vi "Pod Code.vi"() -> ()   [LabVIEW 2017]
uses:
  Type Defs/Relays.ctl
  Type Defs/tempReadings.ctl
  Sensors/Power Sensor - Adafruit INA219/INA219 Measurements.ctl
  Type Defs/telemetryReading.ctl
  <vilib>/Utility/RT CPU Load.ctl
  Type Defs/PodState.ctl
  Type Defs/tofReading.ctl
  Type Defs/pressureReading.ctl
  Type Defs/allLaserReadings.ctl
  Type Defs/laserReading.ctl
  Type Defs/AnalogPressureReading.ctl
  Type Defs/criticalTelemetry.ctl
  Sensors/Time of Flight - VL6180/VL6180 Resource.ctl
  Sensors/Power Sensor - Adafruit INA219/INA219 Config Options.ctl
  Type Defs/thermopileSettings.ctl
  Sensors/Pressure Sensor - BMP180/BMP180 Config Options.ctl
  Type Defs/SensorStates.ctl
  Type Defs/allData.ctl
  <vilib>/Platform/TimedLoop/XDataNode/timing_clust.ctl
  <vilib>/Platform/TimedLoop/XDataNode/nitl_modes.ctl
  <vilib>/Platform/TimedLoop/XDataNode/wakeup.ctl
  <vilib>/myRIO/Instrument Drivers/Onboard IO/DIO/typedefs/DIO Reference.ctl
  <vilib>/myRIO/Common/Instrument Driver Framework/Utilities/typedefs/myRIO Generic Hardware Reference.ctl
  <vilib>/myRIO/Common/Instrument Driver Framework/Utilities/typedefs/Hardware Version Enum.ctl
  <vilib>/myRIO/Common/Instrument Driver Framework/Utilities/typedefs/myRIO v1.0 Reference.ctl
  <vilib>/myRIO/Common/Instrument Driver Framework/Utilities/typedefs/Generic FPGA Reference.ctl
  <vilib>/myRIO/Common/Instrument Driver Framework/myRIO v1.0/DIO/typedefs/DIO Channels List.ctl
  <vilib>/myRIO/Common/Instrument Driver Framework/myRIO v1.0/DIO/typedefs/DIO Channels Enum.ctl
  <vilib>/userdefined/High Color/nirio_resource_hc.ctl
  <vilib>/myRIO/Common/Instrument Driver Framework/Utilities/vis/Is FPGA Ref Available.vi
  <vilib>/myRIO/Common/Instrument Driver Framework/myRIO v1.0/DIO/vis/myRIO v1.1 Open DIO.vi
  <vilib>/myRIO/Instrument Drivers/Onboard IO/DIO/vis/Read.vi
  <vilib>/myRIO/Instrument Drivers/Onboard IO/DIO/vis/Write.vi
  <vilib>/myRIO/Common/Instrument Driver Framework/Utilities/vis/Validate Channels.vi
  <vilib>/myRIO/Common/Instrument Driver Framework/myRIO v1.0/DIO/vis/myRIO v1.0 Reserve DIO.vi
  <vilib>/myRIO/Common/Instrument Driver Framework/myRIO v1.0/Resource Manager/vis/myRIO v1.0 Reserve Channel List.vi
  <vilib>/myRIO/Common/Instrument Driver Framework/myRIO v1.0/DIO/vis/myRIO v1.0 Build MUX Configuration DIO.vi
  <vilib>/myRIO/Common/Instrument Driver Framework/myRIO v1.0/Resource Manager/vis/myRIO v1.0 Reserve Channel.vi
  <vilib>/myRIO/Common/Instrument Driver Framework/myRIO v1.0/Resource Manager/vis/myRIO v1.0 Unreserve Channel.vi
  <vilib>/myRIO/Common/Instrument Driver Framework/myRIO v1.0/Resource Manager/vis/myRIO v1.0 Create Configuration List.vi
  <vilib>/myRIO/Common/Instrument Driver Framework/myRIO v1.0/Resource Manager/vis/myRIO v1.0 Build Mutex Name.vi
  <vilib>/Utility/VariantDataType/GetNumericInfo.vi
  <vilib>/Utility/error.llb/Error Cluster From Error Code.vi
  <vilib>/myRIO/Common/Instrument Driver Framework/myRIO v1.0/myRIO v1.1 Open.vi
  <vilib>/myRIO/Common/Instrument Driver Framework/Utilities/vis/IO Manager.vi
  <vilib>/myRIO/Common/Instrument Driver Framework/Utilities/vis/Configuration Manager.vi
  <vilib>/myRIO/Common/Instrument Driver Framework/myRIO v1.0/Resource Manager/vis/myRIO v1.0 Configure IO.vi
  <vilib>/myRIO/Common/Instrument Driver Framework/myRIO v1.0/myRIO v1.0 Close.vi
  <vilib>/myRIO/Common/Instrument Driver Framework/myRIO v1.0/DIO/vis/myRIO v1.0 Write DIO.vi
  <vilib>/myRIO/Common/Instrument Driver Framework/myRIO v1.0/DIO/vis/myRIO v1.0 Read DIO.vi
  <vilib>/myRIO/Express VI/Onboard IO/DO/DO Express VI.xnode
  <vilib>/myRIO/Instrument Drivers/Onboard IO/DIO/vis/myRIO DIO Open.xnode
  <vilib>/platform/TimedLoop/XDataNode/XDataNode.xnode
  <vilib>/myRIO/Express VI/Onboard IO/DI/DI Express VI.xnode
  <vilib>/myRIO/Instrument Drivers/Onboard IO/DIO/DIO.lvlib
  <vilib>/Platform/TimedLoop/XDataNode/XDNodeRunTimeDep.lvlib
  <vilib>/NI_Real-Time Target Support.lvlib
panel:
  out "Data Snap Period":u32
  out "Slow Sensor Period":u32
  out "State Machine Period":u32
  out "Fast Sensor Period":u32
  out "Actuators":u32
  out "Latest Critical Telemetry":T1
  out "Analog Pressure Reading":T3
  out "Laser Error":errorcluster
  out "Laser Readings":T4
  out "Pressure Reading":T6
  out "ToF Readings":T7[](array[typedef])
  out "Pod State":T2
  in  "Logging":bool
  out "Sensor Error 2":errorcluster
  out "# elements in queue":i32
  out "CPU loads":T8[](array[typedef]) {"ISR (%)" format="%#.2f"; "Idle (%)" format="%#.2f"; "Background (%)" format="%#.2f"; "Normal (%)" format="%#.2f"; "Above Normal (%)" format="%#.2f"; "High (%)" format="%#.2g"; "Timed Structures (%)" format="%#.2g"; "Time Critical (%)" format="%#.2g"; "Total (%)" format="%#.2g"}
  out "Log":T9[][](array[typedef])
  in  "Power I2C Addrs":u8[](array[numeric])=[68, 65, 69] format="%.0x"
  out "Power Readings":T10[](array[typedef]) {"Current" format="%#.3g A"; "Power" format="%#.3g W"; "Shunt Voltage" format=" %#.3g V"; "Bus Voltage" format="%#.3g V"; "Voltage (Total)" format="%#.3g V"}
  out "ThermalReadings":T11[](array[typedef]) {"Ambient Temp (°F)" format="%.2f °F"; "Ambient Temp (°C)" format="%.2f °C"; "Object Temp (°F)" format="%.2f °F"; "Object Temp (°C)" format="%.2f °C"}
  in  "Thermal I2C Addrs":u8[](array[numeric])=[64, 67] format="%.0x"
  in  "Reset Count":bool
  in  "ToFs in use":T12[](array[typedef])=[enum."ToF1", enum."ToF2", enum."ToF3", enum."ToF4"]
  out "Sensor Error":errorcluster
  in  "Reset Sensors":bool
  out "State Error":errorcluster
  in  "Stop Button":bool
  # "Config"
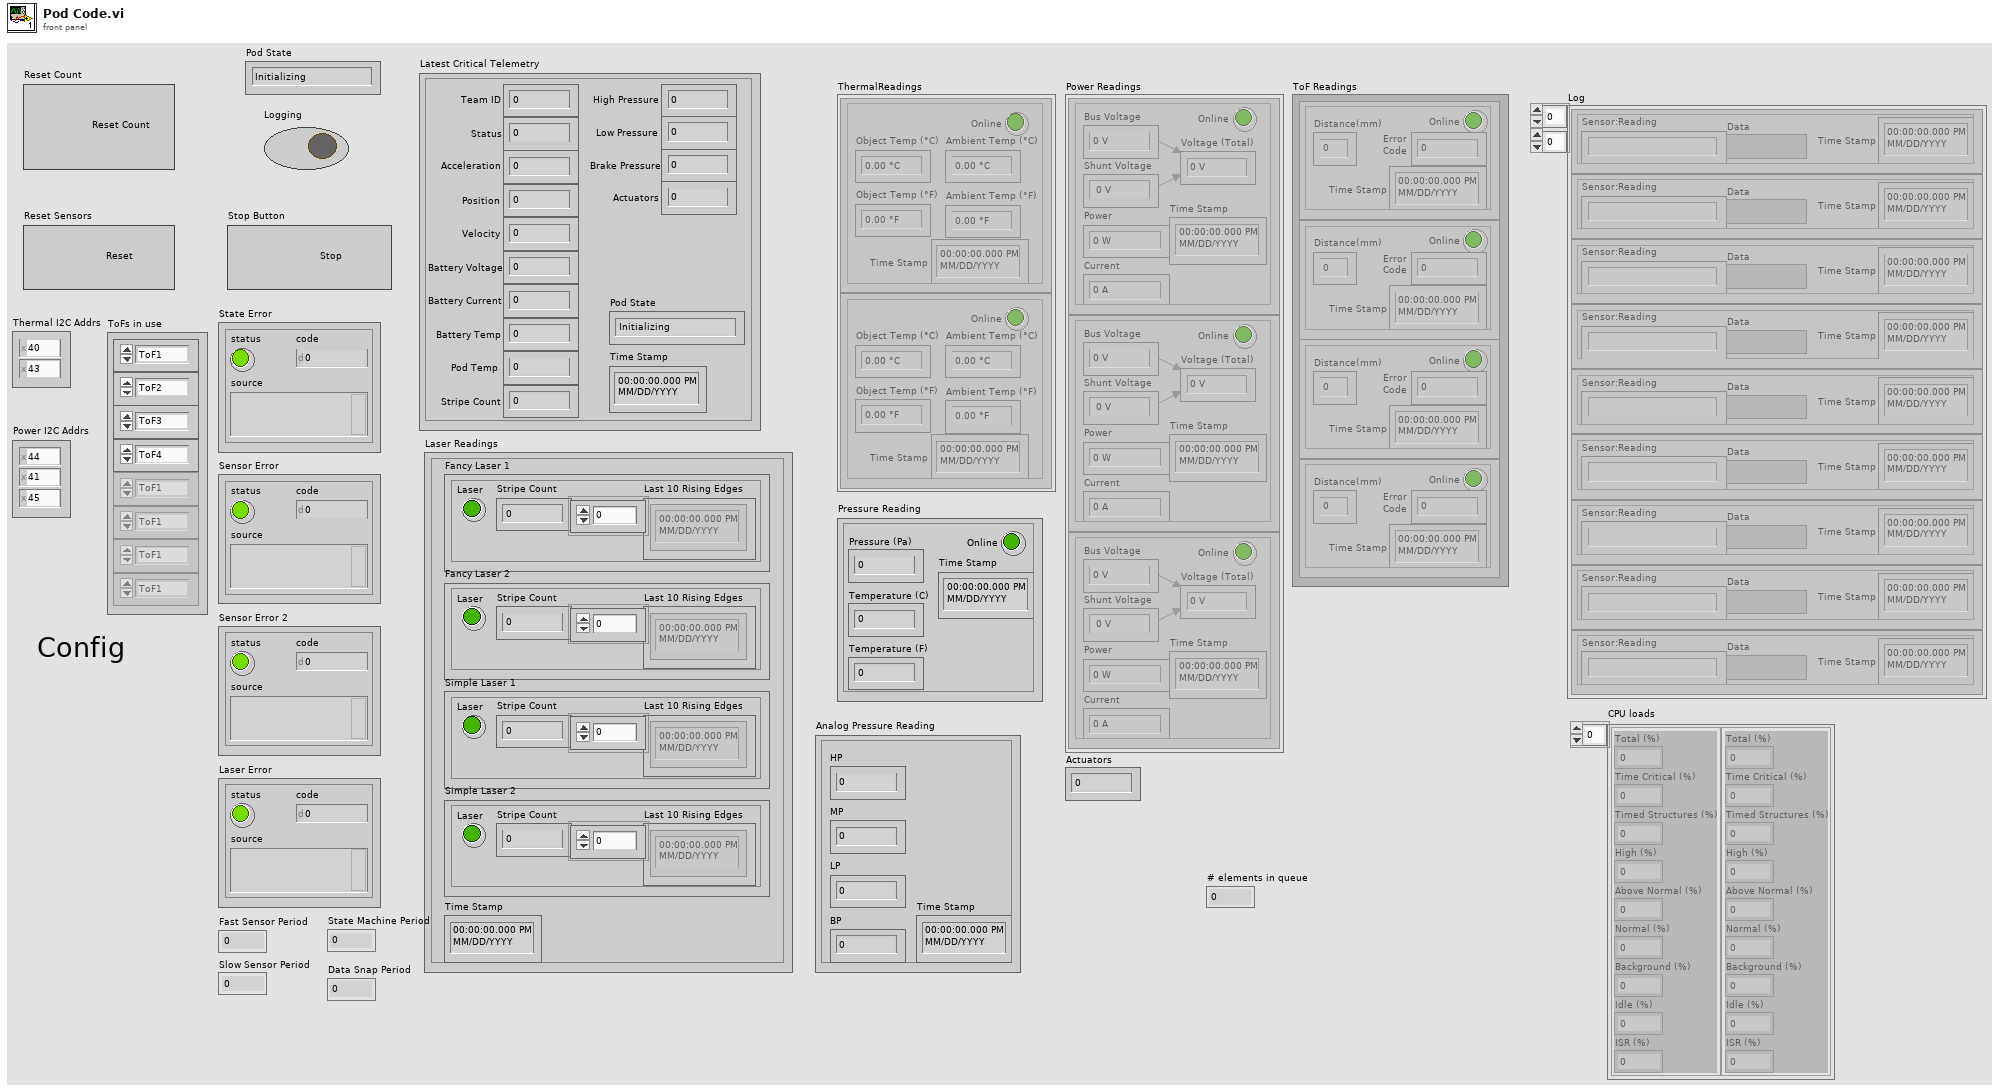
[diagram p1: front panel]
types:
  T1 = typedef "criticalTelemetry.ctl" = cluster{"Team ID":u8, "Status":u8, "Acceleration":i32, "Position":i32, "Velocity":i32, "Battery Voltage":i32, "Battery Current":i32, "Battery Temp":i32, "Pod Temp":i32, "Stripe Count":u32, "High Pressure":dbl, "Low Pressure":dbl, "Brake Pressure":dbl, "Actuators":u32, "Pod State":T2, "Time Stamp":timestamp}
  T2 = typedef "PodState.ctl" = enum16{"Initializing", "Pre-flight Testing", "Ready", "Pushing", "Coast", "Braking", "Post-flight", "Fault"}
  T3 = typedef "AnalogPressureReading.ctl" = cluster{"HP":dbl, "MP":dbl, "LP":dbl, "BP":dbl, "Time Stamp":timestamp}
  T4 = typedef "allLaserReadings.ctl" = cluster{"Fancy Laser 1":T5, "Fancy Laser 2":T5, "Simple Laser 1":T5, "Simple Laser 2":T5, "Time Stamp":timestamp}
  T5 = typedef "laserReading.ctl" = cluster{"Laser":bool, "Stripe Count":u32, "Last 10 Rising Edges":timestamp[]}
  T6 = typedef "pressureReading.ctl" = cluster{"Time Stamp":timestamp, "Online":bool, "Temperature (C)":dbl, "Pressure (Pa)":dbl, "Temperature (F)":dbl}
  T7 = typedef "tofReading.ctl" = cluster{"Distance(mm)":u8, "Online":bool, "Error\nCode":u8, "Time Stamp":timestamp}
  T8 = typedef "NI_Real-Time Target Support.lvlib/RT CPU Load.ctl" = cluster{"Total (%)":dbl, "Time Critical (%)":dbl, "Timed Structures (%)":dbl, "High (%)":dbl, "Above Normal (%)":dbl, "Normal (%)":dbl, "Background (%)":dbl, "Idle (%)":dbl, "ISR (%)":dbl}
  T9 = typedef "telemetryReading.ctl" = cluster{"Sensor:Reading":string, "Data":variant, "Time Stamp":timestamp}
  T10 = typedef "INA219 Measurements.ctl" = cluster{"Voltage (Total)":dbl, "Bus Voltage":dbl, "Shunt Voltage":dbl, "Power":dbl, "Current":dbl, "Online":bool, "Time Stamp":timestamp}
  T11 = typedef "tempReadings.ctl" = cluster{"Object Temp (°C)":dbl, "Object Temp (°F)":dbl, "Ambient Temp (°C)":dbl, "Ambient Temp (°F)":dbl, "Online":bool, "Time Stamp":timestamp}
  T12 = typedef "Relays.ctl" = enum16{"ToF1", "ToF2", "ToF3", "ToF4", "ToF5", "ToF6", "ToF7", "ToF8", "SensePwr", "All"}
  T13 = typedef "SensorStates.ctl" = enum16{"Reset", "Read", "Close"}
  T14 = typedef "BMP180 Config Options.ctl" = cluster{"I2C":cluster{"Slave Address":u8, "Channel":u8}, "Mode":enum8{"Ultra Low Power", "Standard", "High Resolution", "Ultra High Resolution"}, "Cal Coefs":cluster{"AC1":cluster{"Addr:":u8, "Val:":u16}, "AC2":cluster{"Addr:":u8, "Val:":u16}, "AC3":cluster{"Addr:":u8, "Val:":u16}, "AC4":cluster{"Addr:":u8, "Val:":u16}, "AC5":cluster{"Addr:":u8, "Val:":u16}, "AC6":cluster{"Addr:":u8, "Val:":u16}, "B1":cluster{"Addr:":u8, "Val:":u16}, "B2":cluster{"Addr:":u8, "Val:":u16}, "MB":cluster{"Addr:":u8, "Val:":u16}, "MC":cluster{"Addr:":u8, "Val:":u16}, "MD":cluster{"Addr:":u8, "Val:":u16}}, "Online":bool}
  T15 = typedef "thermopileSettings.ctl" = cluster{"Online":bool, "I2C Channel":u8, "I2C Slave Address":u8, "Valid Sample":bool, "Samples to Average":u16, "Last Temp Readings":T11, "Last Reading Time":dbl, "Last Conv Time":dbl}
  T16 = typedef "INA219 Config Options.ctl" = cluster{"I2C":cluster{"Slave Address":u8, "Channel":u8}, "Reset bit":u8, "Bus Voltage Range":u8, "PGA/Shunt Voltage Gain":u8, "Bus Voltage ADC Settings":u8, "Shunt Voltage ADC Settings":u8, "Mode":u8, "Calibration Value":u16, "Online":bool, "Shunt Resistor":dbl}
  T17 = typedef "VL6180 Resource.ctl" = cluster{"I2C Channel":u8, "I2C Slave Address":u8, "Online":bool}
  T18 = typedef "XDNodeRunTimeDep.lvlib/timing_clust.ctl" = cluster{"Expected End [f-1]":u64, "Actual End [f-1]":u64, "Finished Late? [f-1]":bool, "Expected End [i-1]":u64, "Actual End [i-1]":u64, "Finished Late? [i-1]":bool, "Expected Start [i]":u64, "Actual Start [i]":u64, "Expected Start [f]":u64, "Actual Start [f]":u64, "Source Name":string, "Structure Name":string, "Period":i64, "Deadline":i64, "Offset":i64, "Start":i64, "Priority":i32, "Timeout":i32, "Mode":T19, "Wakeup Reason":T20, "Error":errorcluster, "Source Type":string, "Secondary Source Type":string, "Global End Time":u64, "Global Start Time":u64, "Frame Duration":u64, "Iteration Duration":u64, "Assigned CPU":i32, "I/O Scan Engine Mode":u32}
  T19 = typedef "XDNodeRunTimeDep.lvlib/nitl_modes.ctl" = enum32{"No Change", "Process missed periods, maintain original phase", "Discard missed periods, maintain original phase", "Process missed periods, ignore original phase", "Discard missed periods, ignore original phase"}
  T20 = typedef "XDNodeRunTimeDep.lvlib/wakeup.ctl" = enum32{"Normal", "Aborted", "Asynchronous wakeup", "Timing source error", "Timed loop error", "Timeout"}
  T21 = typedef "DIO.lvlib/DIO Reference.ctl" = cluster{"myRIO Reference":T22, "DIO Channels List":T26}
  T22 = typedef "myRIO Generic Hardware Reference.ctl" = cluster{"myRIO Model":T23, "myRIO Hardware Reference":T24}
  T23 = typedef "Hardware Version Enum.ctl" = enum16{"Unknown", "myRIO-1900", "myRIO-1950", "roboRIO", "NI ELVIS RIO CM"}
  T24 = typedef "myRIO v1.0 Reference.ctl" = cluster{"Generic FPGA Reference":T25, "Allow multiple opens":bool}
  T25 = typedef "Generic FPGA Reference.ctl" = refnum<k20>
  T26 = typedef "DIO Channels List.ctl" = T27[]
  T27 = typedef "DIO Channels Enum.ctl" = enum16{"Not Connected", "C/DIO0", "C/DIO1", "C/DIO2", "C/DIO3", "C/DIO4", "C/DIO5", "C/DIO6", "C/DIO7", "A/DIO0", "A/DIO1", "A/DIO2", "A/DIO3", "A/DIO4", "A/DIO5", "A/DIO6", "A/DIO7", "A/DIO8", "A/DIO9", "A/DIO10", "A/DIO11", "A/DIO12", "A/DIO13", "A/DIO14", "A/DIO15", "B/DIO0", "B/DIO1", "B/DIO2", "B/DIO3", "B/DIO4", "B/DIO5", "B/DIO6", "B/DIO7", "B/DIO8", "B/DIO9", "B/DIO10", "B/DIO11", "B/DIO12", "B/DIO13", "B/DIO14", "B/DIO15", "LED0", "LED1", "LED2", "LED3", "Button0", "DIO/DIO0", "DIO/DIO1", "DIO/DIO2", "DIO/DIO3", "DIO/DIO4", "DIO/DIO5", "DIO/DIO6", "DIO/DIO7", "DIO/DIO8", "DIO/DIO9", "SPI/CS0", "SPI/CS1", "SPI/CS2", "SPI/CS3", "LED RADIO (Green)", "LED RADIO (Red)", "LED COMM (Green)", "LED COMM (Red)", "LED MODE (Green)", "LED MODE (Red)"}
  T28 = typedef "nirio_resource_hc.ctl" = tag
  T29 = typedef "allData.ctl" = cluster{"Power Readings":T10[], "ThermalReadings":T11[], "Analog Pressure Reading":T3, "Laser Readings":T4, "Pod State":T2, "seconds since 1Jan1904":timestamp, "ToF Readings":T7[], "CPU loads":T8[], "Actuators":u32, "Pressure Reading":T6, "Laser Error":errorcluster, "Sensor Error":errorcluster, "Sensor Error 2":errorcluster, "State Error":errorcluster}
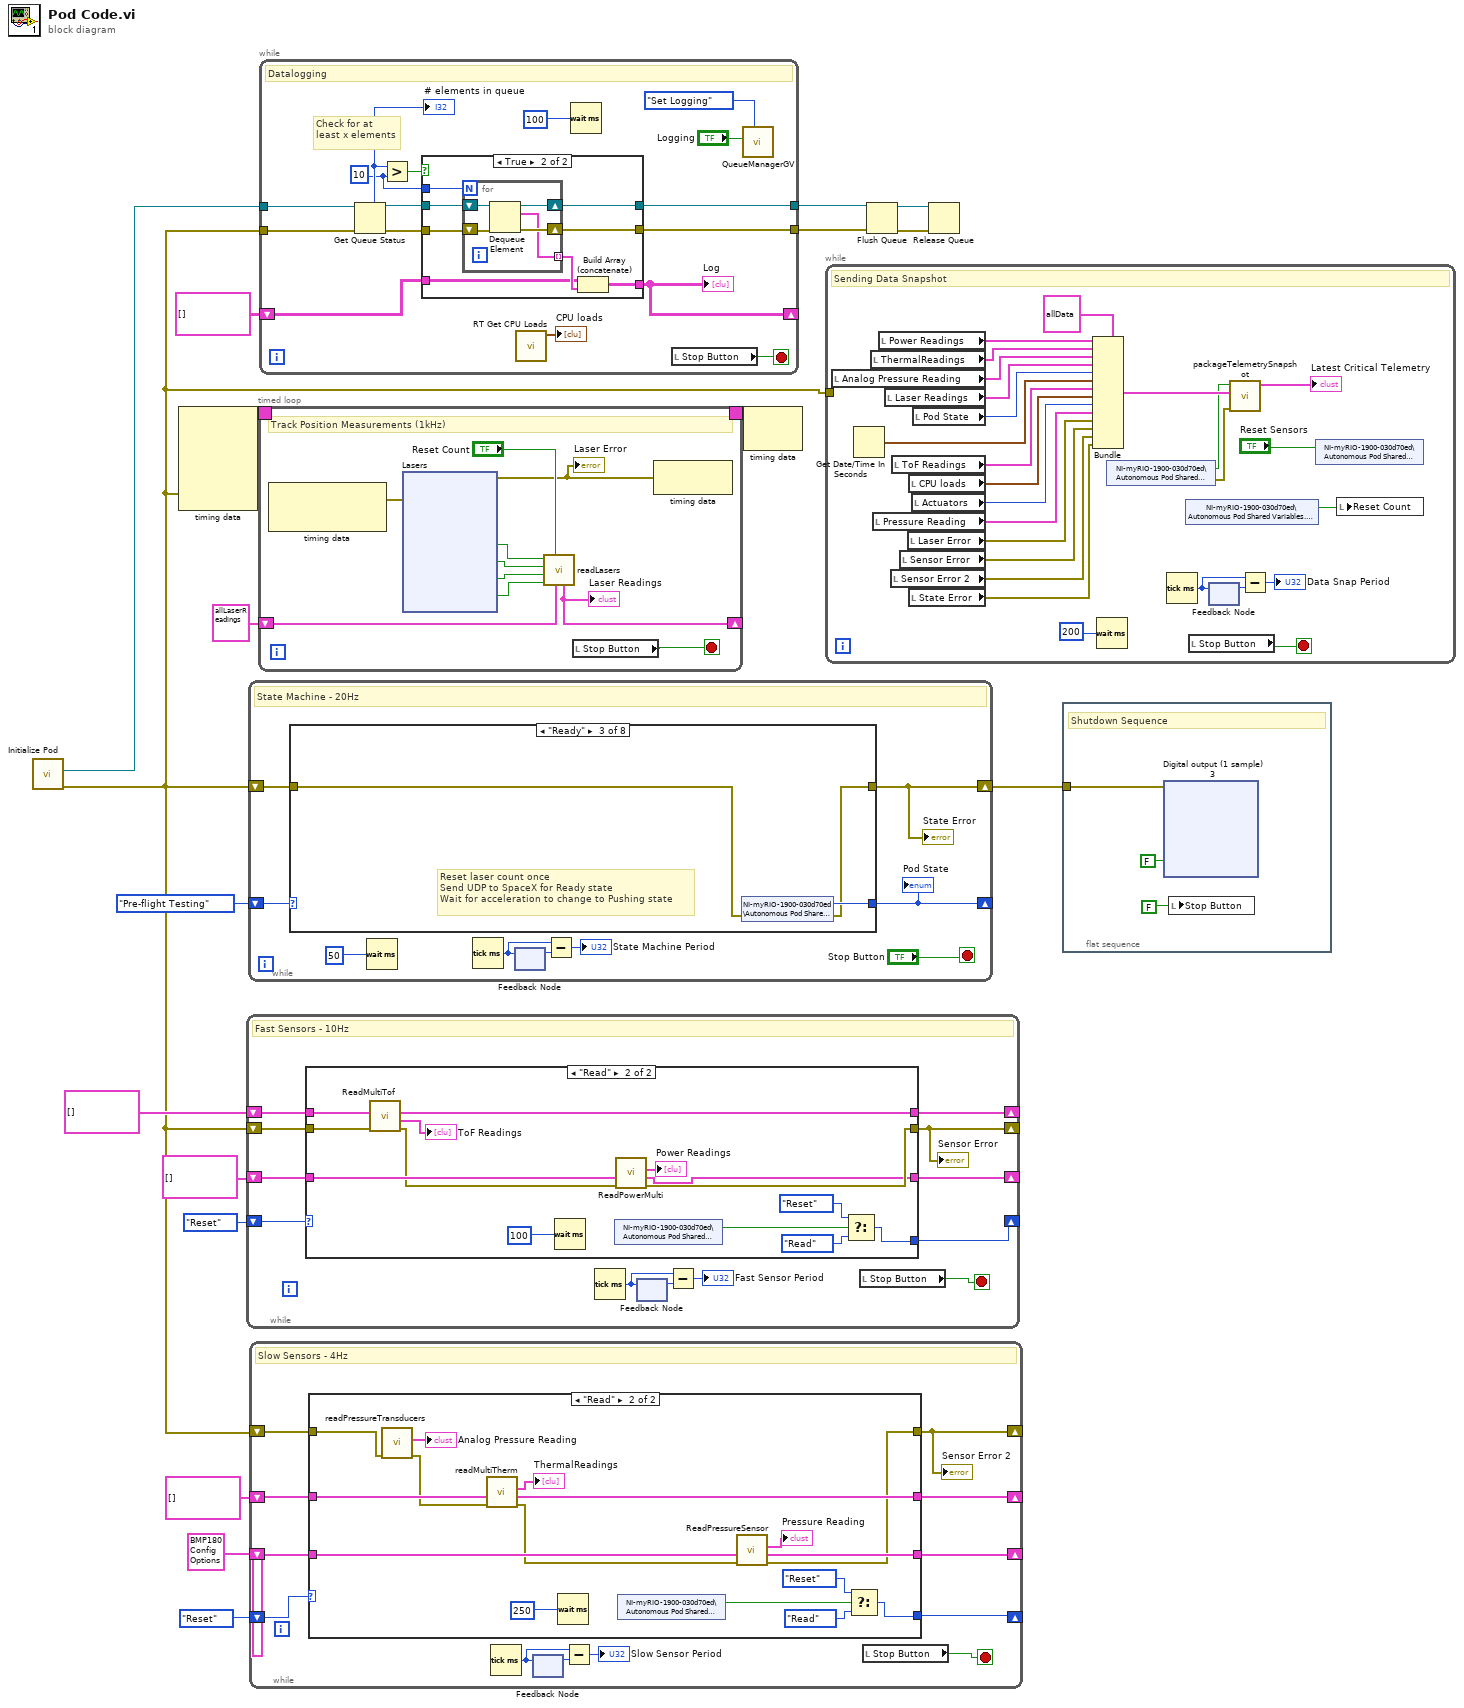
[diagram p0: block diagram]
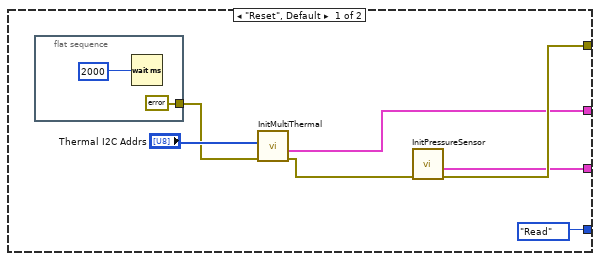
[diagram p3: hidden frame]
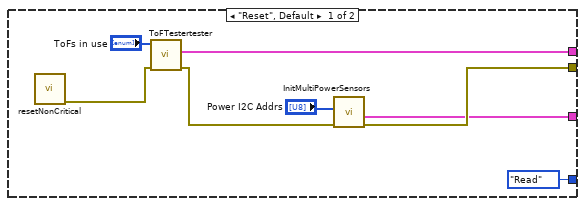
[diagram p4: hidden frame]
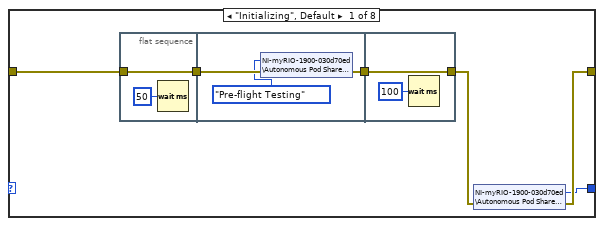
[diagram p5: hidden frame]
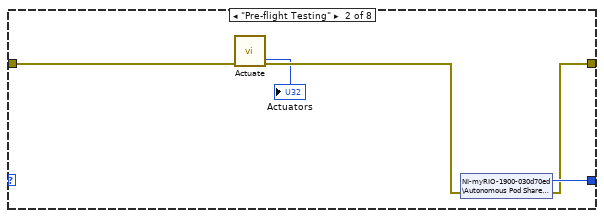
[diagram p6: hidden frame]
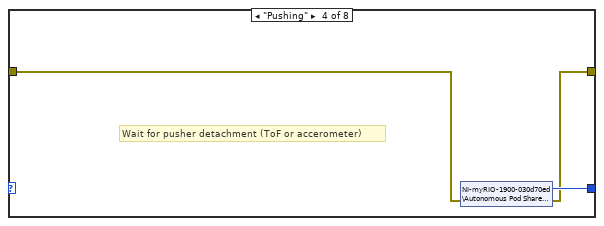
[diagram p7: hidden frame]
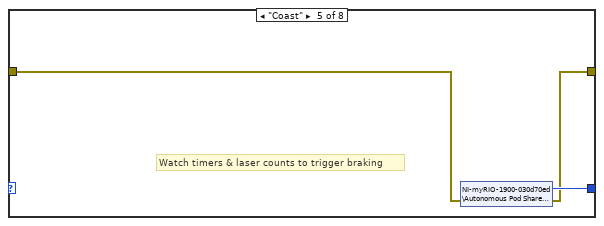
[diagram p8: hidden frame]
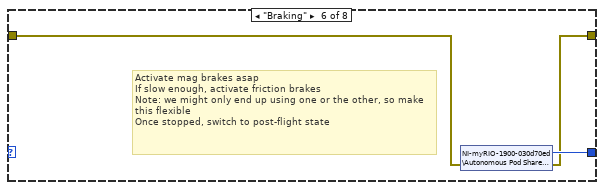
[diagram p9: hidden frame]
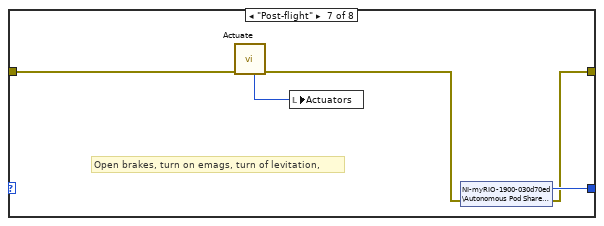
[diagram p10: hidden frame]
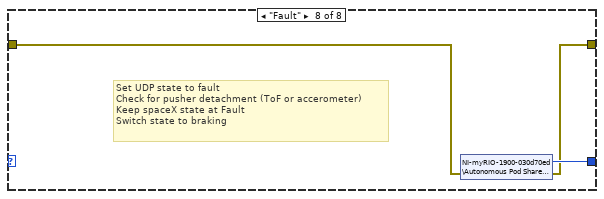
[diagram p11: hidden frame]
diagram:
  n1 = call "Initialize Pod.vi"() -> ("error out"=w2:errorcluster, "Telemetry Queue"=w15:refnum<queue>)  [unwired: 10 in]
  n2 = node-c288(w2) -> (w9:T18)  [unwired: 4 in]
  n3 = while {
    shift-right: [w28] -> _
    shift-left: SensorStates."Reset" -> [w30]
    shift-right: [w24] -> _
    shift-left: w2 -> [w29]
    shift-right: [w26] -> _
    shift-left: T17[] [] ("VL Configs") -> [w25]
    shift-right: [w19] -> _
    shift-left: T16[] [] ("Config Out") -> [w23]
    stop <- w27 stop-if-true
    # "Fast Sensors - 10Hz"
    n4 = case shown="\"Read\"" w30 {
      tunnel: w29 -> [_ w47]
      tunnel: [w34 w42] -> w24
      tunnel: [SensorStates."Read" w51] -> w28
      tunnel: [w31 w46] -> w26
      tunnel: w25 -> [_ w48]
      tunnel: w23 -> [_ w44]
      tunnel: [w32 w39] -> w19
      frame "Reset", Default {
        n5 = call "resetNonCritical.vi"() -> ("error out"=w37:errorcluster)  [unwired: 11 in]
        n6 = call "ToFTestertester.vi"("error in"=w37, "ToFs"="ToFs in use") -> ("error out"=w33:errorcluster, "ToF Details"=w31:T17[])  [unwired: 7 in, 1 out]
        n7 = call "InitMultiPowerSensors.vi"("error in"=w33, "I2C Addresses"="Power I2C Addrs") -> ("error out"=w34:errorcluster, "Power Sensors Configs"=w32:T16[])  [unwired: 7 in, 1 out]
      }
      frame "Read" {
        n8 = call "ReadMultiTof.vi"("error in"=w47, "VL6180 Resources"=w48) -> ("error out"=w41:errorcluster, "ToF Readings"=→"ToF Readings":T7[], "VL Configs"=w46:T17[])  [unwired: 6 in, 1 out]
        n9 = Wait (ms)(milliseconds to wait=u32 100) -> ()  [unwired: 1 out]
        n10 = shared-variable "NI-myRIO-1900-030d70ed\\Autonomous Pod Shared Variables.lvlib\\ResetSensor"() -> (w45:bool)  [unwired: 1 in, 1 out]
        n11 = call "ReadPowerMulti.vi"("error in"=w41, "Config In"=w44) -> ("error out"=w42:errorcluster, "Config Out"=w39:T16[], "Power Readings"=→"Power Readings":T10[])  [unwired: 7 in]
        n12 = Select(t=SensorStates."Reset", s=w45, f=SensorStates."Read") -> (s? t:f=w51:T13)
      }
    }
    "Sensor Error" <- w24
    n13 = Tick Count (ms)() -> (millisecond timer value=w21:u32)
    n14 = feedback-in #1(w21) -> ()
    n15 = feedback #1() -> (w22:u32)  [unwired: 1 in]
    n16 = Subtract(x=w21, y=w22) -> (x-y=→"Fast Sensor Period":u32)
    n17 = local read "Stop Button"() -> (w27:bool)
  }
  n18 = while {
    shift-right: [w57] -> w13
    shift-left: w2 -> [w59]
    shift-right: [w56] -> _
    shift-left: PodState."Pre-flight Testing" ("Pod States") -> [w58]
    stop <- "Stop Button" stop-if-true
    # "State Machine - 20Hz"
    n19 = case shown="\"Ready\"" w58 {
      tunnel: w59 -> [w67 w77 w80 w83 w86 w89 w94 w97]
      tunnel: [w63 w78 w81 w84 w87 w90 w95 w98] -> w57
      tunnel: [w62 w79 w82 w85 w88 w91 w96 w99] -> w56
      frame "Initializing", Default {
        n20 = flat-sequence {
          tunnel: w67 -> [w68]
          tunnel: [w68] -> w66
          tunnel: w66 -> [w72]
          tunnel: [w71] -> w64
          tunnel: [w73] -> w65
          tunnel: w64 -> [w73]
          frame #0 {
            n21 = Wait (ms)(milliseconds to wait=u32 50) -> ()  [unwired: 1 out]
          }
          frame #1 {
            n22 = shared-variable "NI-myRIO-1900-030d70ed\\Autonomous Pod Shared Variables.lvlib\\PodState"(PodState."Pre-flight Testing" ("Pod States"), error in=w72) -> (error out=w71:errorcluster)
          }
          frame #2 {
            n23 = Wait (ms)(milliseconds to wait=u32 100) -> ()  [unwired: 1 out]
          }
        }
        n24 = shared-variable "NI-myRIO-1900-030d70ed\\Autonomous Pod Shared Variables.lvlib\\PodState"(error in=w65) -> (w62:T2, error out=w63:errorcluster)
      }
      frame "Pre-flight Testing" {
        n25 = call "Actuate.vi"("error in"=w77) -> ("error out"=w76:errorcluster, "Actuators"=→"Actuators":u32)  [unwired: 8 in, 1 out]
        n26 = shared-variable "NI-myRIO-1900-030d70ed\\Autonomous Pod Shared Variables.lvlib\\PodState"(error in=w76) -> (w79:T2, error out=w78:errorcluster)
      }
      frame "Ready" {
        # "Reset laser count once\nSend UDP to SpaceX for Ready state\nWait for acceleration to change to Pushing state"
        n27 = shared-variable "NI-myRIO-1900-030d70ed\\Autonomous Pod Shared Variables.lvlib\\PodState"(error in=w80) -> (w82:T2, error out=w81:errorcluster)
      }
      frame "Pushing" {
        # "Wait for pusher detachment (ToF or accerometer)"
        n28 = shared-variable "NI-myRIO-1900-030d70ed\\Autonomous Pod Shared Variables.lvlib\\PodState"(error in=w83) -> (w85:T2, error out=w84:errorcluster)
      }
      frame "Coast" {
        # "Watch timers & laser counts to trigger braking"
        n29 = shared-variable "NI-myRIO-1900-030d70ed\\Autonomous Pod Shared Variables.lvlib\\PodState"(error in=w86) -> (w88:T2, error out=w87:errorcluster)
      }
      frame "Braking" {
        # "Activate mag brakes asap\nIf slow enough, activate friction brakes\nNote: we might only end up using one or the other, so make this flexible\nOnce stopped, switch to post-flight state"
        n30 = shared-variable "NI-myRIO-1900-030d70ed\\Autonomous Pod Shared Variables.lvlib\\PodState"(error in=w89) -> (w91:T2, error out=w90:errorcluster)
      }
      frame "Post-flight" {
        # "Open brakes, turn on emags, turn of levitation,"
        n31 = call "Actuate.vi"("error in"=w94) -> ("error out"=w93:errorcluster, "Actuators"=w92:u32)  [unwired: 8 in, 1 out]
        n32 = local write "Actuators"(w92) -> ()
        n33 = shared-variable "NI-myRIO-1900-030d70ed\\Autonomous Pod Shared Variables.lvlib\\PodState"(error in=w93) -> (w96:T2, error out=w95:errorcluster)
      }
      frame "Fault" {
        # "Set UDP state to fault\nCheck for pusher detachment (ToF or accerometer)\nKeep spaceX state at Fault\nSwitch state to braking"
        n34 = shared-variable "NI-myRIO-1900-030d70ed\\Autonomous Pod Shared Variables.lvlib\\PodState"(error in=w97) -> (w99:T2, error out=w98:errorcluster)
      }
    }
    "State Error" <- w57
    "Pod State" <- w56
    n35 = Wait (ms)(milliseconds to wait=u32 50) -> ()  [unwired: 1 out]
    n36 = Tick Count (ms)() -> (millisecond timer value=w53:u32)
    n37 = feedback #2() -> (w54:u32)  [unwired: 1 in]
    n38 = feedback-in #2(w53) -> ()
    n39 = Subtract(x=w53, y=w54) -> (x-y=→"State Machine Period":u32)
  }
  n40 = while {
    shift-right: [w109] -> _
    shift-left: SensorStates."Reset" -> [w111]
    shift-right: [w107] -> _
    shift-left: w2 -> [w110]
    shift-right: [w106] -> _
    shift-left: T15[] [] ("ThermalConfigs") -> [w105]
    shift-right: [w104] -> _
    shift-left: T14 {"I2C"={"Slave Address"=64, "Channel"=0}, "Mode"=enum."Ultra Low Power", "Cal Coefs"={"AC1"={"Addr:"=170, "Val:"=0}, "AC2"={"Addr:"=172, "Val:"=0}, "AC3"={"Addr:"=174, "Val:"=0}, "AC4"={"Addr:"=176, "Val:"=0}, "AC5"={"Addr:"=178, "Val:"=0}, "AC6"={"Addr:"=180, "Val:"=0}, "B1"={"Addr:"=182, "Val:"=0}, "B2"={"Addr:"=184, "Val:"=0}, "MB"={"Addr:"=186, "Val:"=0}, "MC"={"Addr:"=188, "Val:"=0}, "MD"={"Addr:"=190, "Val:"=0}}, "Online"=FALSE} ("BMP180 Config Options") -> [w103]
    stop <- w108 stop-if-true
    # "Slow Sensors - 4Hz"
    n41 = case shown="\"Read\"" w111 {
      tunnel: w110 -> [_ w124]
      tunnel: [w117 w127] -> w107
      tunnel: [SensorStates."Read" w135] -> w109
      tunnel: [w112 w131] -> w106
      tunnel: w105 -> [_ w130]
      tunnel: [w114 w128] -> w104
      tunnel: w103 -> [_ w129]
      frame "Reset", Default {
        n42 = flat-sequence {
          tunnel: [errorcluster {"status"=FALSE, "code"=0, "source"=""} ("error in")] -> w113
          frame #0 {
            n43 = Wait (ms)(milliseconds to wait=u32 2000) -> ()  [unwired: 1 out]
          }
        }
        n44 = call "InitMultiThermal.vi"("error in"=w113, "I2C Addresses"="Thermal I2C Addrs") -> ("error out"=w115:errorcluster, "ThermalConfigs"=w112:T15[])  [unwired: 6 in, 2 out]
        n45 = call "InitPressureSensor.vi"("error in"=w115) -> ("error out"=w117:errorcluster, "BMP180 Config Options"=w114:T14)  [unwired: 9 in]
      }
      frame "Read" {
        n46 = call "readPressureTransducers.vi"("error in"=w124) -> ("error out"=w123:errorcluster, "Analog Pressure Reading"=→"Analog Pressure Reading":T3)  [unwired: 9 in]
        n47 = call "readMultiTherm.vi"("error in"=w123, "ThermalConfigs"=w130) -> ("error out"=w125:errorcluster, "ThermalConfigs"=w131:T15[], "ThermReadings"=→"ThermalReadings":T11[])  [unwired: 6 in, 1 out]
        n48 = Wait (ms)(milliseconds to wait=u32 250) -> ()  [unwired: 1 out]
        n49 = shared-variable "NI-myRIO-1900-030d70ed\\Autonomous Pod Shared Variables.lvlib\\ResetSensor"() -> (w132:bool)  [unwired: 1 in, 1 out]
        n50 = call "ReadPressureSensor.vi"("error in (no error)"=w125, "BMP180 Config Options"=w129) -> ("error out"=w127:errorcluster, "BMP180 Config"=w128:T14, "Pressure Reading"=→"Pressure Reading":T6)  [unwired: 7 in]
        n51 = Select(t=SensorStates."Reset", s=w132, f=SensorStates."Read") -> (s? t:f=w135:T13)
      }
    }
    "Sensor Error 2" <- w107
    n52 = Tick Count (ms)() -> (millisecond timer value=w100:u32)
    n53 = feedback #3() -> (w102:u32)  [unwired: 1 in]
    n54 = feedback-in #3(w100) -> ()
    n55 = Subtract(x=w100, y=w102) -> (x-y=→"Slow Sensor Period":u32)
    n56 = local read "Stop Button"() -> (w108:bool)
  }
  n57 = timed-loop {
    timing: w9 -> [_]
    timing-out: [_] -> w8
    shift-right: [w138] -> _
    shift-left: T4 {"Fancy Laser 1"={"Laser"=FALSE, "Stripe Count"=0, "Last 10 Rising Edges"=[]}, "Fancy Laser 2"={"Laser"=FALSE, "Stripe Count"=0, "Last 10 Rising Edges"=[]}, "Simple Laser 1"={"Laser"=FALSE, "Stripe Count"=0, "Last 10 Rising Edges"=[]}, "Simple Laser 2"={"Laser"=FALSE, "Stripe Count"=0, "Last 10 Rising Edges"=[]}, "Time Stamp"=timestamp(0 s since 1904-01-01)} ("Laser Readings") -> [w137]
    stop <- w146 stop-if-true
    # "Track Position Measurements (1kHz)"
    n58 = node-c288() -> (w144:errorcluster)  [unwired: 1 in, 1 out]
    n59 = xnode "Lasers"("error in (no error)"=w144) -> ("Fancy Laser 1 (B/DIO11 (Pin 18))"=w141:bool, "Fancy Laser 2 (A/DIO7 (Pin 25))"=w139:bool, "Laser 1 (B/DIO9 (Pin 29))"=w142:bool, "Laser 2 (B/DIO10 (Pin 31))"=w140:bool, "error out"=w143:errorcluster)
    "Laser Error" <- w143
    n60 = call "readLasers.vi"("Laser Readings In"=w137, "Reset Count"="Reset Count", "Simple Laser 2"=w140, "Simple Laser 1"=w142, "Fancy Laser 2"=w139, "Fancy Laser 1"=w141) -> ("Laser Readings"=w138:T4)  [unwired: 5 in]
    "Laser Readings" <- w138
    n61 = local read "Stop Button"() -> (w146:bool)
    n62 = node-c288(w143) -> ()  [unwired: 1 out]
  }
  n63 = while {
    tunnel: w2 -> [w204]
    tunnel: w15 -> [w202]
    tunnel: [w197] -> w5
    tunnel: [w196] -> w4
    shift-right: [w195] -> _
    shift-left: T9[][] [] -> [w194]
    stop <- w205 stop-if-true
    w200 = 10 ("y")
    # "Check for at least x elements"
    # "Datalogging"
    n64 = Get Queue Status(queue=w202, error in (no error)=w204) -> (queue out=w199:refnum<queue>, error out=w198:errorcluster, # elements in queue=w203:i32)  [unwired: 1 in, 5 out]
    "# elements in queue" <- w203
    n65 = Greater?(x=w203, y=w200) -> (0:w201:bool)
    n66 = case shown="True" w201 {
      tunnel: w200 -> [_ w216]
      tunnel: w199 -> [w208 w215]
      tunnel: w198 -> [w207 w214]
      tunnel: [w208 w213] -> w197
      tunnel: [w207 w212] -> w196
      tunnel: [w206 w209] -> w195
      tunnel: w194 -> [w206 w210]
      frame False {
      }
      frame True {
        n67 = for {
          N: w216 -> [_]
          shift-right: [w219] -> w213
          shift-left: w215 -> [w221]
          shift-right: [w218] -> w212
          shift-left: w214 -> [w220]
          tunnel: [w217] -> w211 mode=indexing
          n68 = Dequeue Element(queue=w221, error in (no error)=w220) -> (queue out=w219:refnum<queue>, element=w217:T9, error out=w218:errorcluster)  [unwired: 1 in, 1 out]
        }
        n69 = Build Array (concatenate)(w210, w211) -> (w209:T9[][])
      }
    }
    "Log" <- w195
    n70 = call <vilib>:"RT Get CPU Loads.vi"() -> ("CPU loads"=→"CPU loads":T8[])  [unwired: 10 in, 1 out]
    n71 = Wait (ms)(milliseconds to wait=u32 100) -> ()  [unwired: 1 out]
    n72 = local read "Stop Button"() -> (w205:bool)
    n73 = call "QueueManagerGV.vi"("Command"=enum16{"Get", "Set Logging", "Set Queue"}."Set Logging", "Logging"="Logging") -> ()  [unwired: 8 in, 2 out]
  }
  n74 = node-c288(w8) -> ()  [unwired: 1 out]
  n75 = while {
    tunnel: w2 -> [_]
    stop <- w247 stop-if-true
    # "Sending Data Snapshot"
    n76 = local read "Analog Pressure Reading"() -> (w243:T3)
    n77 = Get Date/Time In Seconds() -> (seconds since 1Jan1904=w240:timestamp)
    n78 = local read "ThermalReadings"() -> (w244:T11[])
    n79 = local read "Pressure Reading"() -> (w236:T6)
    n80 = local read "Power Readings"() -> (w245:T10[])
    n81 = local read "Laser Readings"() -> (w242:T4)
    n82 = local read "Sensor Error 2"() -> (w233:errorcluster)
    n83 = local read "ToF Readings"() -> (w239:T7[])
    n84 = local read "Sensor Error"() -> (w234:errorcluster)
    n85 = local read "Laser Error"() -> (w235:errorcluster)
    n86 = local read "CPU loads"() -> (w238:T8[])
    n87 = local read "State Error"() -> (w232:errorcluster)
    n88 = local read "Actuators"() -> (w237:u32)
    n89 = local read "Pod State"() -> (w241:T2)
    n90 = Bundle(cluster=T29 {"Power Readings"=[{"Voltage (Total)"=0.0, "Bus Voltage"=0.0, "Shunt Voltage"=0.0, "Power"=0.0, "Current"=0.0, "Online"=FALSE, "Time Stamp"=timestamp(0 s since 1904-01-01)}, {"Voltage (Total)"=13.1728, "Bus Voltage"=13.148, "Shunt Voltage"=0.024800000000000003, "Power"=3.1746448000000003, "Current"=0.24100000000000002, "Online"=TRUE, "Time Stamp"=timestamp(2082864055.371957 s since 1904-01-01)}, {"Voltage (Total)"=24.13995, "Bus Voltage"=24.14, "Shunt Voltage"=-5e-05, "Power"=-0.002413995, "Current"=-0.0001, "Online"=TRUE, "Time Stamp"=timestamp(2082864055.374175 s since 1904-01-01)}], "ThermalReadings"=[{"Object Temp (°C)"=23.0625, "Object Temp (°F)"=73.5125, "Ambient Temp (°C)"=24.09375, "Ambient Temp (°F)"=75.36875, "Online"=TRUE, "Time Stamp"=timestamp(2082864055.392536 s since 1904-01-01)}, {"Object Temp (°C)"=22.84375, "Object Temp (°F)"=73.11875, "Ambient Temp (°C)"=24.0625, "Ambient Temp (°F)"=75.3125, "Online"=TRUE, "Time Stamp"=timestamp(2082864055.394416 s since 1904-01-01)}], "Analog Pressure Reading"={"HP"=-248.613281392, "MP"=-248.613281392, "LP"=-248.959961044, "BP"=-248.613281392, "Time Stamp"=timestamp(2082864055.390519 s since 1904-01-01)}, "Laser Readings"={"Fancy Laser 1"={"Laser"=FALSE, "Stripe Count"=0, "Last 10 Rising Edges"=[]}, "Fancy Laser 2"={"Laser"=FALSE, "Stripe Count"=0, "Last 10 Rising Edges"=[]}, "Simple Laser 1"={"Laser"=FALSE, "Stripe Count"=0, "Last 10 Rising Edges"=[]}, "Simple Laser 2"={"Laser"=TRUE, "Stripe Count"=0, "Last 10 Rising Edges"=[]}, "Time Stamp"=timestamp(2082864055.32697 s since 1904-01-01)}, "Pod State"=enum."Pre-flight Testing", "seconds since 1Jan1904"=timestamp(2082864055.398343 s since 1904-01-01), "ToF Readings"=[{"Distance(mm)"=51, "Online"=TRUE, "Error\nCode"=0, "Time Stamp"=timestamp(2082864055.298114 s since 1904-01-01)}, {"Distance(mm)"=12, "Online"=TRUE, "Error\nCode"=0, "Time Stamp"=timestamp(2082864055.317715 s since 1904-01-01)}, {"Distance(mm)"=9, "Online"=TRUE, "Error\nCode"=0, "Time Stamp"=timestamp(2082864055.335987 s since 1904-01-01)}, {"Distance(mm)"=25, "Online"=TRUE, "Error\nCode"=0, "Time Stamp"=timestamp(2082864055.353802 s since 1904-01-01)}], "CPU loads"=[{"Total (%)"=78.03635031413472, "Time Critical (%)"=0.0, "Timed Structures (%)"=0.32081374652993544, "High (%)"=0.0, "Above Normal (%)"=0.0, "Normal (%)"=76.33465617759227, "Background (%)"=0.0, "Idle (%)"=21.963649685865278, "ISR (%)"=1.3808803900125173}, {"Total (%)"=56.1031514616488, "Time Critical (%)"=0.0, "Timed Structures (%)"=21.009799080061946, "High (%)"=0.0, "Above Normal (%)"=0.0, "Normal (%)"=34.915435601607804, "Background (%)"=0.0, "Idle (%)"=43.8968485383512, "ISR (%)"=0.17791677997904956}], "Actuators"=14848, "Pressure Reading"={"Time Stamp"=timestamp(0 s since 1904-01-01), "Online"=FALSE, "Temperature (C)"=0.0, "Pressure (Pa)"=0.0, "Temperature (F)"=0.0}, "Laser Error"={"status"=FALSE, "code"=0, "source"=""}, "Sensor Error"={"status"=FALSE, "code"=0, "source"=""}, "Sensor Error 2"={"status"=FALSE, "code"=0, "source"=""}, "State Error"={"status"=FALSE, "code"=0, "source"=""}} ("All Data"), "Power Readings"=w245, "ThermalReadings"=w244, "Analog Pressure Reading"=w243, "Laser Readings"=w242, "Pod State"=w241, "seconds since 1Jan1904"=w240, "ToF Readings"=w239, "CPU loads"=w238, "Actuators"=w237, "Pressure Reading"=w236, "Laser Error"=w235, "Sensor Error"=w234, "Sensor Error 2"=w233, "State Error"=w232) -> (w231:T29)
    n91 = Wait (ms)(milliseconds to wait=u32 200) -> ()  [unwired: 1 out]
    n92 = shared-variable "NI-myRIO-1900-030d70ed\\Autonomous Pod Shared Variables.lvlib\\sendNcData"() -> (w227:bool, error out=w228:errorcluster)  [unwired: 1 in]
    n93 = Tick Count (ms)() -> (millisecond timer value=w226:u32)
    n94 = shared-variable "NI-myRIO-1900-030d70ed\\Autonomous Pod Shared Variables.lvlib\\ResetLaserCount"() -> (w222:bool)  [unwired: 1 in, 1 out]
    n95 = local read "Stop Button"() -> (w247:bool)
    n96 = feedback #4() -> (w225:u32)  [unwired: 1 in]
    n97 = feedback-in #4(w226) -> ()
    n98 = call "packageTelemetrySnapshot.vi"("Error In"=w228, "All Data"=w231, "Send Non-Critical Data"=w227) -> ("Latest Critical Telemetry"=→"Latest Critical Telemetry":T1)  [unwired: 7 in, 1 out]
    n99 = Subtract(x=w226, y=w225) -> (x-y=→"Data Snap Period":u32)
    n100 = shared-variable "NI-myRIO-1900-030d70ed\\Autonomous Pod Shared Variables.lvlib\\ResetSensor"("Reset Sensors") -> ()  [unwired: 1 in, 1 out]
    n101 = local write "Reset Count"(w222) -> ()
  }
  n102 = Flush Queue(queue=w5, error in (no error)=w4) -> (queue out=w6:refnum<queue>, error out=w7:errorcluster)  [unwired: 1 out]
  n103 = Release Queue(queue=w6, error in (no error)=w7) -> ()  [unwired: 1 in, 3 out]
  n104 = flat-sequence {
    tunnel: w13 -> [w248]
    frame #0 {
      # "Shutdown Sequence"
      n105 = xnode "Digital output (1 sample) 3"("Activate Pneumatics (A/DIO10 (Pin 31))"=FALSE ("Levitation"), "error in (no error)"=w248) -> ()  [unwired: 1 out]
      n106 = local write "Stop Button"(FALSE ("Stop Button")) -> ()
    }
  }
